vi "Substitute Actor.vi"(10 "Substitute Actor in":refnum<class "Actor.lvclass">, 11 "Current Command Actor":refnum<class "Command Actor.lvclass">) -> (0 "error out":errorcluster, 2 "Substitute Actor out":refnum<class "Actor.lvclass">)   [LabVIEW 2014, in "Robot Actor Framework.lvlib" / "Command Actor.lvlib" / "Command Actor.lvclass"]
doc: "(<B>Filename</B>: Actor Framework.lvlib:Actor.lvclass:Substitute Actor.vi)\n\nThis method copies information from the <b>Current Actor</b> to the <b>Substitute Actor</b>, including the to-self and the to-caller queue references. The purpose of this function is to allow an actor to define a method that replaces itself with another actor, useful for implementing a State Pattern Actor. Child classes should override this method to copy any additional fields that they need from the current to the substitute.\n\nThis method may return error code 678010: Illegal substitution. Overrides of this method may choose to return this error if the new actor is not one that is an appropriate substitute for the current actor, for whatever standards of \"appropriate\" are chosen for the current actor. If returning an error, override VIs should return the unmodified <b>Current Actor</b> as <b>Substitute Actor out</b>."
uses:
  Command Actor.lvclass
  <vilib>/ActorFramework/Actor/Actor.lvclass
  Command Actor.lvclass/Command Actor.ctl
  <vilib>/ni/Actors/State Actor/State Actor/State Actor.lvclass
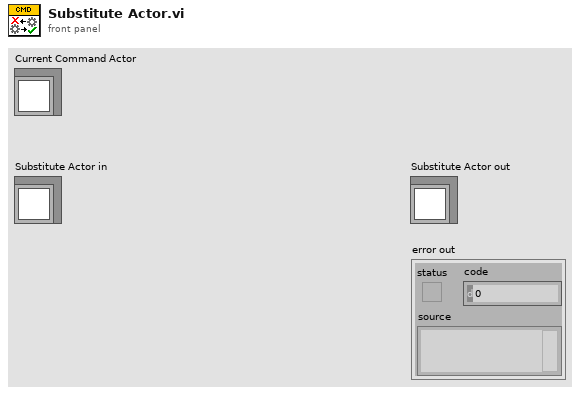
[diagram p1: front panel]
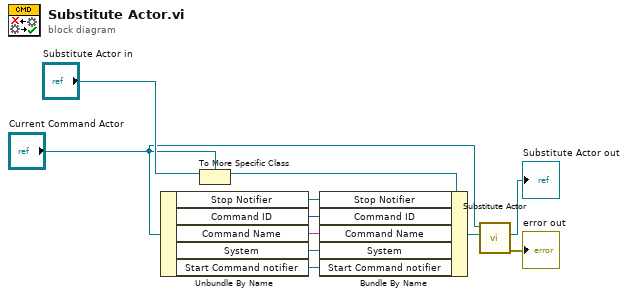
[diagram p0: block diagram]
diagram:
  n1 = Unbundle By Name("Current Command Actor") -> ("Stop Notifier"=w6:refnum<notifier>, "Command ID"=w5:u32, "Command Name"=w4:string, "System"=w2:refnum<class "Message Enqueuer.lvclass">, "Start Command notifier"=w1:refnum<notifier>)
  n2 = To More Specific Class(target class="Current Command Actor", reference="Substitute Actor in") -> (specific class reference=w8:refnum<class "Command Actor.lvclass">)  [unwired: 1 in, 1 out]
  n3 = Bundle By Name(cluster=w8, "Stop Notifier"=w6, "Command ID"=w5, "Command Name"=w4, "System"=w2, "Start Command notifier"=w1) -> (w7:refnum<class "Command Actor.lvclass">)
  n4 = call-parent "Substitute Actor.vi"("Substitute Actor in"=w7, "Current Actor"="Current Command Actor") -> ("error out"=→"error out":errorcluster, "Substitute Actor out"=→"Substitute Actor out":refnum<class "Actor.lvclass">)  [unwired: 8 in]
